vi "LW_ChooseCorrectInstrument.vi"(3 "Instrument Keys":string[](array[string]), 5 "error in (no error)":errorcluster) -> (16 "selected instrument key":string, 19 "error out":errorcluster)   [LabVIEW 2015]
panel:
  in  "select\nmy instrument":bool
  in  "Instrument Keys List":u16(ring) items=["CONEX-CC (A6U1PBW3)"]
  # "If you have instruments connected but still the list is blank, then \ncross-check if the \"Newport.CONEXAGAP.CommandInterface.DLL\" \nis linked to your constructor node as per the document."
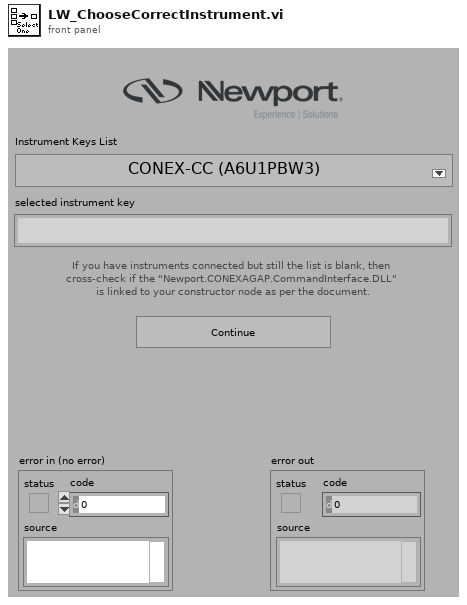
[diagram p1: front panel]
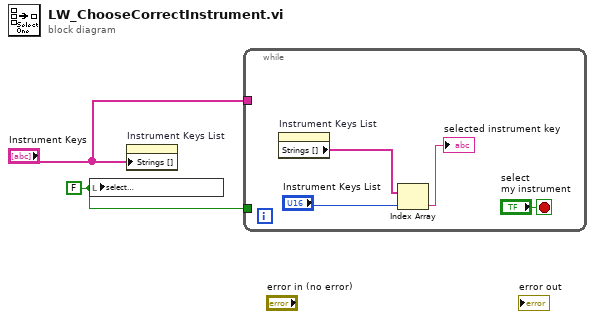
[diagram p0: block diagram]
diagram:
  w1 = FALSE ("stop")
  n1 = local write "select\nmy instrument"(w1) -> ()
  n2 = property on="Instrument Keys List" class="Ring (strict)"("Strings []"="Instrument Keys") -> ()  [unwired: 2 in, 2 out]
  n3 = while {
    tunnel: "Instrument Keys" -> [_]
    tunnel: w1 -> [_]
    stop <- "select\nmy instrument" stop-if-true
    n4 = property on="Instrument Keys List" class="Ring (strict)"() -> ("Strings []"=w5:string[])  [unwired: 2 in, 2 out]
    n5 = Index Array(array=w5, index="Instrument Keys List") -> (element=→"selected instrument key":string)
  }
